vi "HandleError.vi"(8 "error in (no error)":errorcluster, 11 "SimpleErrorLogger in":refnum<class "SimpleErrorLogger.lvclass">) -> (0 "error out":errorcluster, 3 "SimpleErrorLogger out":refnum<class "SimpleErrorLogger.lvclass">)   [LabVIEW 2023, in "SimpleErrorLogger.lvlib" / "SimpleErrorLogger.lvclass"]
uses:
  SimpleErrorLogger.lvclass
  SimpleErrorLogger.lvclass/SimpleErrorLogger.ctl
  <vilib>/ActorFramework/Actor/Actor.lvclass
  SimpleErrorLogger Messages/LogError Msg/LogError Msg.lvclass
  <vilib>/ActorFramework/Message Enqueuer/Message Priority.ctl
  <vilib>/ActorFramework/Message Enqueuer/Message Enqueuer.lvclass
  C:/Program Files (x86)/National Instruments/LabVIEW 2023/vi.lib/ActorFramework/Actor/Actor.lvclass
  C:/Source/LabVIEW/Error_Logger/SimpleErrorLogger/SimpleErrorLogger/SimpleErrorLogger.lvclass
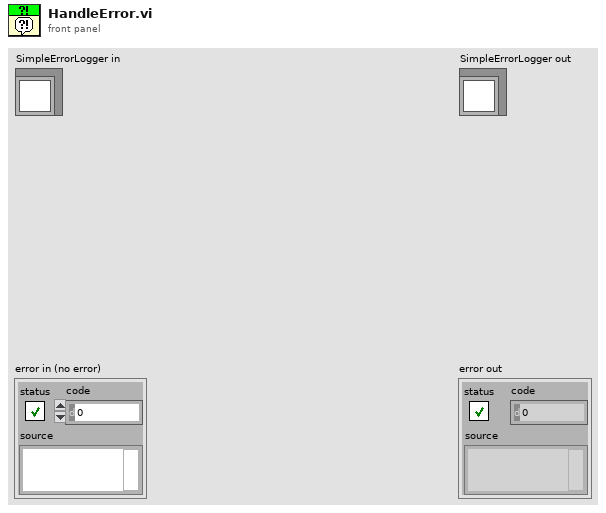
[diagram p1: front panel]
types:
  T1 = typedef "Actor Framework.lvlib/Message Enqueuer.lvclass/Message Priority.ctl" = enum16{"Low", "Normal", "High"}
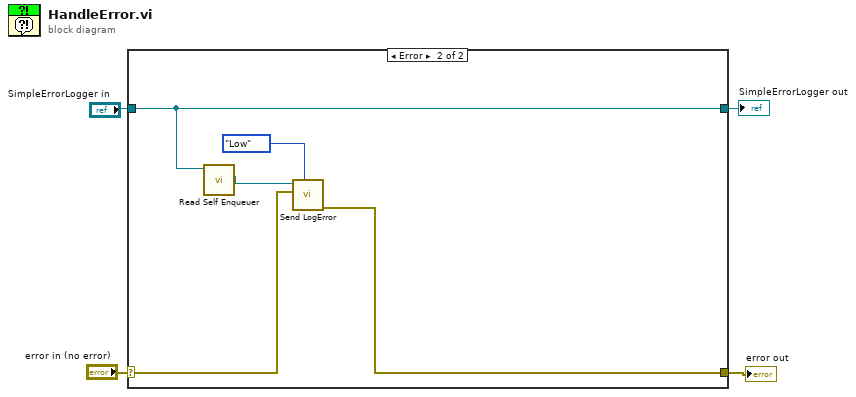
[diagram p0: block diagram]
diagram:
  n1 = case shown="Error" "error in (no error)" {
    selector: "error in (no error)" -> [w5 w9]
    tunnel: [w5 w8] -> w3
    tunnel: [w6 w11] -> w1
    tunnel: "SimpleErrorLogger in" -> [w6 w11]
    frame No Error {
    }
    frame Error {
      n2 = call <vilib>:"Read Self Enqueuer.vi"("Actor"=w11) -> ("Self Enqueuer"=w10:refnum<class "Message Enqueuer.lvclass">)  [unwired: 10 in]
      n3 = call "Send LogError.vi"("Message Priority (Normal)"=Message_Priority."Low", "error"=w9, "Message Enqueuer"=w10) -> ("error out"=w8:errorcluster)  [unwired: 7 in, 1 out]
    }
  }
  "error out" <- w3
  "SimpleErrorLogger out" <- w1
